vi "Write Complex Extended Value.vi"(8 "error in (no error)":errorcluster, 10 "Complex Double Float":cxt[](array[numeric]), 11 "Numeric in":refnum<class "Abs_Extended Float 1D.lvclass">) -> (0 "error out":errorcluster, 3 "Numeric out":refnum<class "Abs_Extended Float 1D.lvclass">)   [LabVIEW 2021, in "Abs_Extended Float 1D.lvclass"]
uses:
  Abs_Extended Float 1D.lvclass
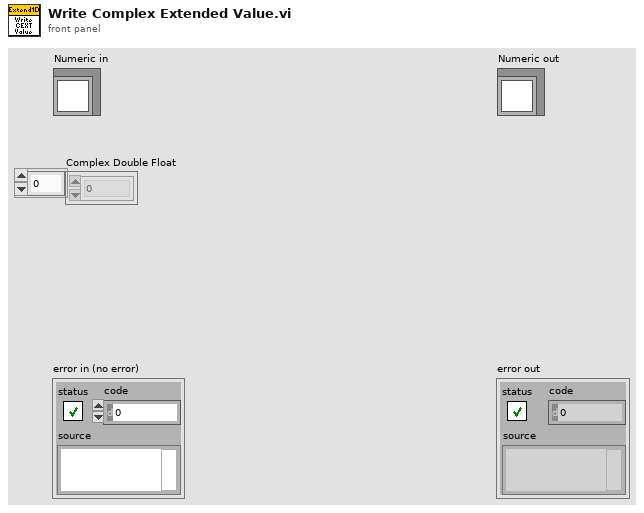
[diagram p1: front panel]
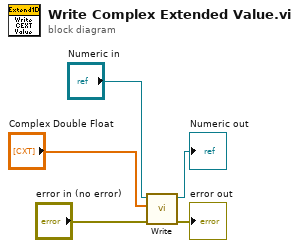
[diagram p0: block diagram]
diagram:
  n1 = call-dynamic "Write.vi"("error in (no error)"="error in (no error)", "Value"="Complex Double Float", "Abs_Extend1D Float.lvclass in"="Numeric in") -> ("error out"=→"error out":errorcluster, "Abs_Extend1D Float.lvclass out"=→"Numeric out":refnum<class "Abs_Extended Float 1D.lvclass">)  [unwired: 7 in]
